vi "runtimeTests.vi"(6 "Tolerance":dbl, 7 "Machine Settings":cluster{"Max Value":dbl, "Min Value":dbl}, 9 "Signal":dbl, 10 "Setpoint":dbl) -> (2 "Danger?":bool)   [LabVIEW 2018]
panel:
  out "_Min Value":dbl
  out "_Max Value":dbl
  # "This is a flat sequence test to determine if machine is operating within specifications"
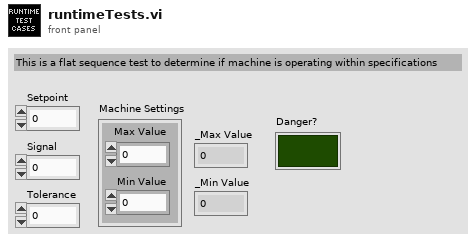
[diagram p1: front panel]
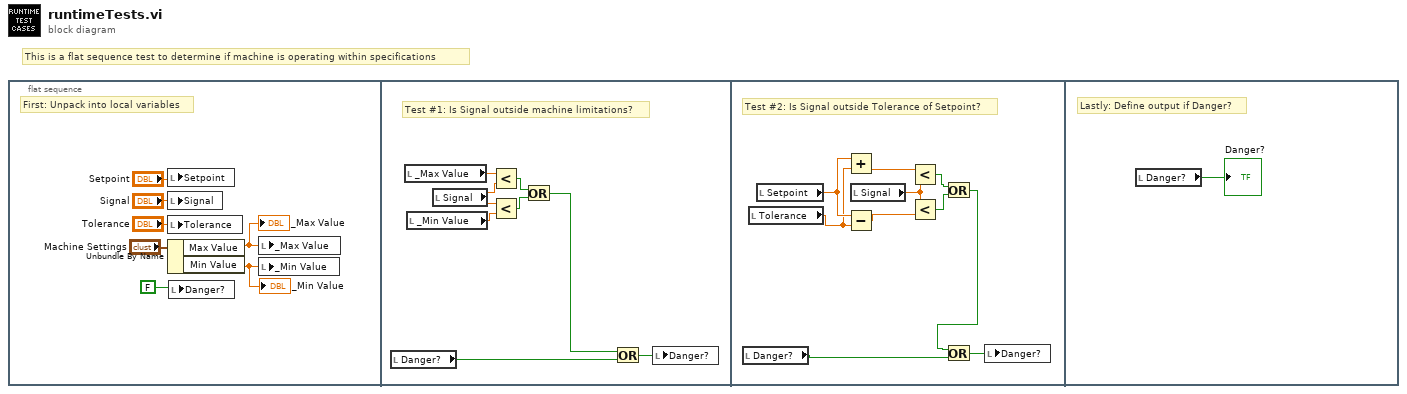
[diagram p0: block diagram]
diagram:
  # "This is a flat sequence test to determine if machine is operating within specifications"
  n1 = flat-sequence {
    frame #0 {
      # "First: Unpack into local variables"
      n2 = local write "Setpoint"("Setpoint") -> ()
      n3 = local write "Signal"("Signal") -> ()
      n4 = local write "Tolerance"("Tolerance") -> ()
      n5 = Unbundle By Name("Machine Settings") -> ("Max Value"=w2:dbl, "Min Value"=w3:dbl)
      "_Min Value" <- w3
      "_Max Value" <- w2
      n6 = local write "Danger?"(FALSE) -> ()
      n7 = local write "_Max Value"(w2) -> ()
      n8 = local write "_Min Value"(w3) -> ()
    }
    frame #1 {
      # "Test #1: Is Signal outside machine limitations?"
      n9 = local read "Danger?"() -> (w10:bool)
      n10 = local read "_Max Value"() -> (w14:dbl)
      n11 = local read "_Min Value"() -> (w15:dbl)
      n12 = local read "Signal"() -> (w13:dbl)
      n13 = Less?(x=w14, y=w13) -> (x < y?=w12:bool)
      n14 = Less?(x=w13, y=w15) -> (x < y?=w11:bool)
      n15 = Or(x=w12, y=w11) -> (x .or. y?=w8:bool)
      n16 = Or(x=w8, y=w10) -> (x .or. y?=w9:bool)
      n17 = local write "Danger?"(w9) -> ()
    }
    frame #2 {
      # "Test #2: Is Signal outside Tolerance of Setpoint?"
      n18 = local read "Danger?"() -> (w24:bool)
      n19 = local read "Tolerance"() -> (w22:dbl)
      n20 = local read "Setpoint"() -> (w23:dbl)
      n21 = Add(x=w23, y=w22) -> (x+y=w19:dbl)
      n22 = Subtract(x=w23, y=w22) -> (x-y=w20:dbl)
      n23 = local read "Signal"() -> (w21:dbl)
      n24 = Less?(x=w19, y=w21) -> (x < y?=w17:bool)
      n25 = Less?(x=w21, y=w20) -> (x < y?=w18:bool)
      n26 = Or(x=w17, y=w18) -> (x .or. y?=w16:bool)
      n27 = Or(x=w16, y=w24) -> (x .or. y?=w25:bool)
      n28 = local write "Danger?"(w25) -> ()
    }
    frame #3 {
      # "Lastly: Define output if Danger?"
      n29 = local read "Danger?"() -> (→"Danger?":bool)
    }
  }
